vi "Ejercicio_19_display_7_segmentos.vi"() -> ()   [LabVIEW 2020]
panel:
  in  "stop 2":bool
  out "Unidades":dbl
  out "Decenas":dbl
  in  "Selector":i32
  out "Centenas":bool
  out "Decenas":bool
  out "Unidades":bool
  out "c":bool
  out "e":bool
  out "b":bool
  out "f":bool
  out "d":bool
  out "g":bool
  out "a":bool
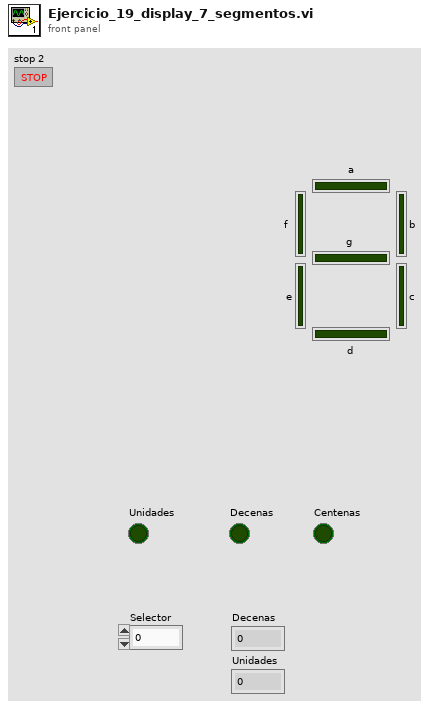
[diagram p1: front panel]
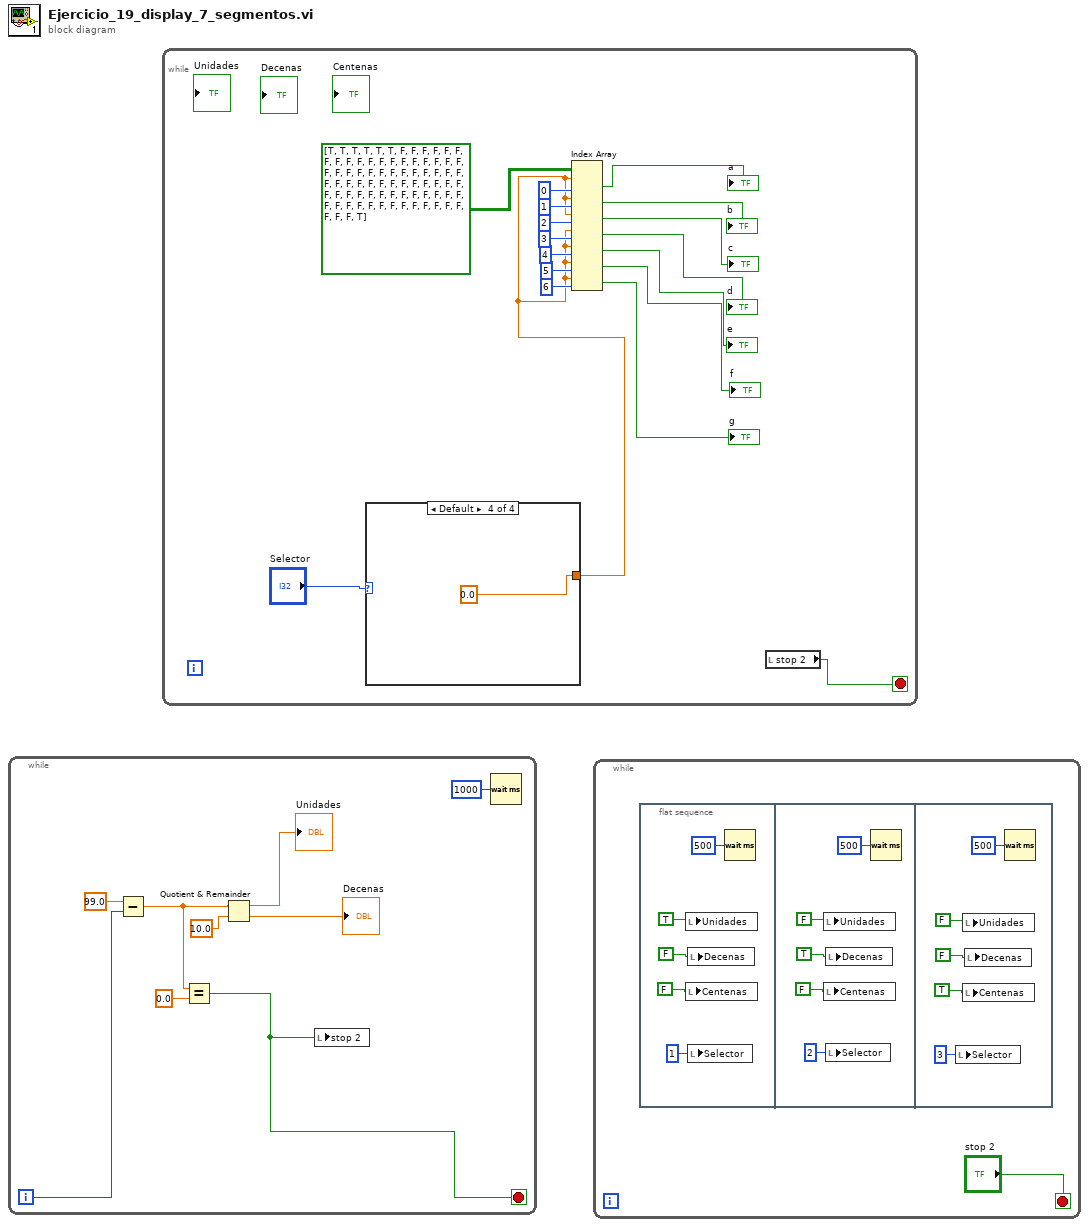
[diagram p0: block diagram]
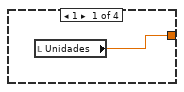
[diagram p2: hidden frame]
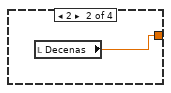
[diagram p3: hidden frame]
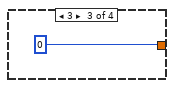
[diagram p4: hidden frame]
diagram:
  n1 = while {
    i -> [w7]
    stop <- w1 stop-if-true
    n2 = Subtract(x=99.0, y=w7) -> (x-y=w5:dbl)
    n3 = Equal?(x=w5, y=0.0) -> (x = y?=w1:bool)
    n4 = Quotient & Remainder(x=w5, y=10.0) -> (x-y*floor(x/y)=→"Unidades":dbl, floor(x/y)=→"Decenas":dbl)
    n5 = local write "stop 2"(w1) -> ()
    n6 = Wait (ms)(milliseconds to wait=u32 1000) -> ()  [unwired: 1 out]
  }
  n7 = while {
    stop <- w10 stop-if-true
    n8 = case shown="Default" "Selector" {
      tunnel: [w28 w29 0 0.0] -> w16
      frame 1 {
        n9 = local read "Unidades"() -> (w28:dbl)
      }
      frame 2 {
        n10 = local read "Decenas"() -> (w29:dbl)
      }
      frame 3 {
      }
      frame Default {
      }
    }
    n11 = Index Array "Index Array"(array=bool[][] [[TRUE, TRUE, TRUE, TRUE, TRUE, TRUE, FALSE, FALSE, FALSE], [FALSE, FALSE, FALSE, FALSE, FALSE, FALSE, FALSE, FALSE, FALSE], [FALSE, FALSE, FALSE, FALSE, FALSE, FALSE, FALSE, FALSE, FALSE], [FALSE, FALSE, FALSE, FALSE, FALSE, FALSE, FALSE, FALSE, FALSE], [FALSE, FALSE, FALSE, FALSE, FALSE, FALSE, FALSE, FALSE, FALSE], [FALSE, FALSE, FALSE, FALSE, FALSE, FALSE, FALSE, FALSE, FALSE], [FALSE, FALSE, FALSE, FALSE, FALSE, FALSE, FALSE, FALSE, FALSE], [FALSE, FALSE, FALSE, FALSE, FALSE, FALSE, FALSE, FALSE, FALSE], [FALSE, FALSE, FALSE, FALSE, FALSE, FALSE, FALSE, FALSE, TRUE]], index (row) #1=w16, index (col) #1=0 ("disabled index (col)"), index (row) #2=w16, index (col) #2=1 ("index (col)"), index (row) #3=w16, index (col) #3=2 ("index (col)"), index (row) #4=w16, index (col) #4=3 ("index (col)"), index (row) #5=w16, index (col) #5=4 ("index (col)"), index (row) #6=w16, index (col) #6=5 ("index (col)"), index (row) #7=w16, index (col) #7=6 ("index (col)")) -> (element #1=→"a":bool, element #2=→"b":bool, element #3=→"c":bool, element #4=→"d":bool, element #5=→"e":bool, element #6=→"f":bool, element #7=→"g":bool)
    n12 = local read "stop 2"() -> (w10:bool)
  }
  n13 = while {
    stop <- "stop 2" stop-if-true
    n14 = flat-sequence {
      frame #0 {
        n15 = local write "Unidades"(TRUE) -> ()
        n16 = local write "Centenas"(FALSE) -> ()
        n17 = local write "Decenas"(FALSE) -> ()
        n18 = local write "Selector"(1 ("Selector")) -> ()
        n19 = Wait (ms)(milliseconds to wait=u32 500) -> ()  [unwired: 1 out]
      }
      frame #1 {
        n20 = local write "Unidades"(FALSE) -> ()
        n21 = local write "Centenas"(FALSE) -> ()
        n22 = local write "Decenas"(TRUE) -> ()
        n23 = local write "Selector"(2 ("Selector")) -> ()
        n24 = Wait (ms)(milliseconds to wait=u32 500) -> ()  [unwired: 1 out]
      }
      frame #2 {
        n25 = local write "Selector"(3 ("Selector")) -> ()
        n26 = local write "Unidades"(FALSE) -> ()
        n27 = local write "Centenas"(TRUE) -> ()
        n28 = local write "Decenas"(FALSE) -> ()
        n29 = Wait (ms)(milliseconds to wait=u32 500) -> ()  [unwired: 1 out]
      }
    }
  }
